vi "runOuterLoopClock.vi"(8 "error in (no error)":errorcluster, 11 "Boot in":refnum<class "Boot.lvclass">) -> (0 "error out":errorcluster, 3 "Boot out":refnum<class "Boot.lvclass">)   [LabVIEW 2016, in "Boot.lvclass"]
uses:
  Boot.lvclass
  Boot.lvclass/Boot.ctl
  UserEvents/UserEvents.lvclass/UserEvents.ctl
  Commands/UpdateCommand/UpdateCommand.lvclass
  D:/Code/ts_M1M3Support/Commands/Command/Command.lvclass
  DataTypes/General/ProcessCommandEvent.ctl
  Commands/Command/Command.lvclass
  Common_RT_FPGA/IIRQ/IIRQ.lvclass
  DataTypes/General/M1M3SupportGeneral.lvlib
  UserEvents/UserEvents.lvclass
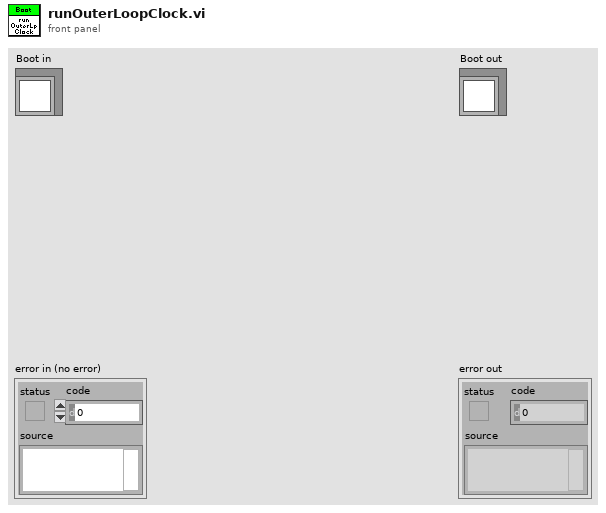
[diagram p1: front panel]
types:
  T1 = typedef "M1M3SupportGeneral.lvlib/ProcessCommandEvent.ctl" = cluster{"Command":refnum<class "Command.lvclass">}
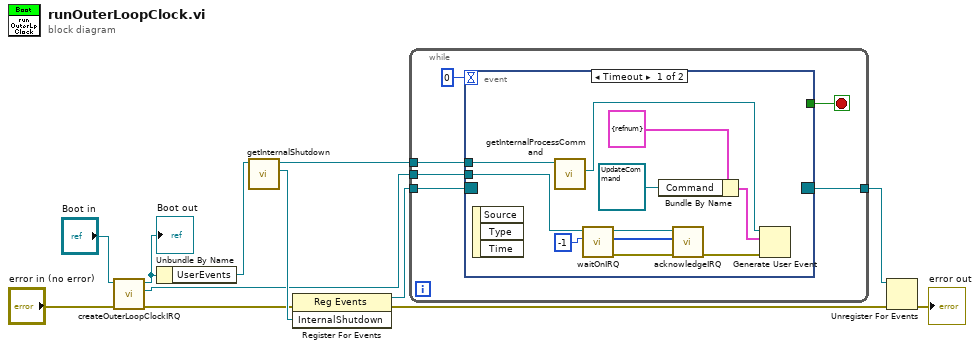
[diagram p0: block diagram]
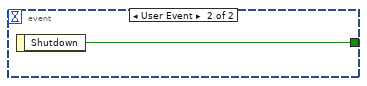
[diagram p2: hidden frame]
diagram:
  n1 = call "createOuterLoopClockIRQ.vi"("error in (no error)"="error in (no error)", "Boot in"="Boot in") -> ("error out"=w3:errorcluster, "OuterLoopClockIRQ"=w6:refnum<class "IIRQ.lvclass">, "Boot out"=w11:refnum<class "Boot.lvclass">)  [unwired: 7 in]
  "Boot out" <- w11
  n2 = Unbundle By Name(w11) -> ("UserEvents"=w9:refnum<class "UserEvents.lvclass">)
  n3 = call "getInternalShutdown.vi"("UserEvents in"=w9) -> ("InternalShutdown"=w8:refnum<user-event>, "UserEvents out"=w5:refnum<class "UserEvents.lvclass">)  [unwired: 9 in]
  n4 = register-events(error in=w3, w8) -> (reference out=w7:refnum<event-registration>, error out=w2:errorcluster)  [unwired: 1 in]
  n5 = while {
    tunnel: w7 -> [w17]
    tunnel: [w16] -> w4
    tunnel: w5 -> [w14]
    tunnel: w6 -> [w13]
    stop <- w15 stop-if-true
    n6 = event shown="[0] Timeout" {
      selector: w17 -> [_ _]
      dyn-events: [_ _] -> w16
      timeout: 0 -> [_ _]
      tunnel: [_ w30] -> w15
      tunnel: w14 -> [w29 _]
      tunnel: w13 -> [w23 _]
      event Timeout {
        n7 = event-data() -> ()  [unwired: 1 in, 3 out]
        n8 = call "getInternalProcessCommand.vi"("UserEvents in"=w29) -> ("InternalProcessCommand"=w25:refnum<user-event>)  [unwired: 9 in, 1 out]
        n9 = call-dynamic "waitOnIRQ.vi"("Timeout"=-1 ("Timeout (ms)"), "IIRQ in"=w23) -> ("error out"=w20:errorcluster, "IRQs"=w22:i32[], "IIRQ out"=w21:refnum<class "IIRQ.lvclass">)  [unwired: 6 in, 1 out]
        n10 = Bundle By Name(cluster=T1 {"Command"=refnum} ("ProcessCommandEvent"), "Command"=refnum<class "UpdateCommand.lvclass"> refnum ("UpdateCommand.lvclass")) -> (w26:T1)
        n11 = call-dynamic "acknowledgeIRQ.vi"("error in (no error)"=w20, "IRQs"=w22, "IIRQ in"=w21) -> ("error out"=w19:errorcluster)  [unwired: 7 in, 1 out]
        n12 = Generate User Event(user event=w25, event data cluster=w26, error in=w19) -> ()  [unwired: 1 in, 2 out]
      }
      event User Event {
        n13 = event-data() -> ("Shutdown"=w30:bool)  [unwired: 1 in]
      }
    }
  }
  n14 = Unregister For Events(event registration refnum=w4, error in=w2) -> (error out=→"error out":errorcluster)
